vi "Redetection_Final EVT OUT.vi"(4 "Sweep # IN":i32, 5 "Detected event (1D)":cluster{dbl[][]}[](array[cluster]), 6 "EVT # (redetected)":i32, 7 "Number of event IN":i32[][](array[numeric])) -> (1 "Final EVT OUT":dbl[][](array[numeric]), 3 "Distribution (output)":T1)   [LabVIEW 2017]
uses:
  <vilib>/Analysis/NI_AALPro.lvlib
  <vilib>/Analysis/NI_AALBase.lvlib
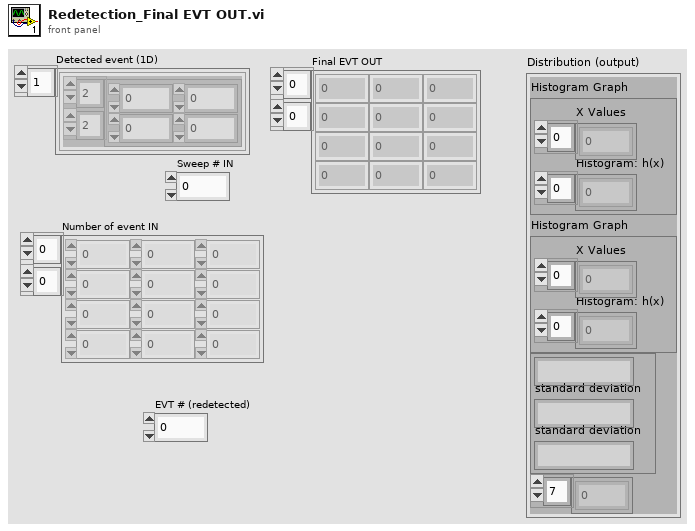
[diagram p1: front panel]
types:
  T1 = cluster{"Histogram Graph":cluster{"X Values":dbl[], "Histogram: h(x)":i32[]}, "Histogram Graph":cluster{"X Values":dbl[], "Histogram: h(x)":i32[]}, cluster{string, "standard deviation":string, "standard deviation":string}, i32[]}
  T2 = cluster{string, "standard deviation":string, "standard deviation":string}
  T3 = cluster{"X Values":dbl[], "Histogram: h(x)":i32[]}
  T4 = cluster{"Histogram Graph":cluster{"X Values":dbl[], "Histogram: h(x)":i32[]}, "Histogram Graph":cluster{"X Values":dbl[], "Histogram: h(x)":i32[]}, cluster{string, "standard deviation":string, "standard deviation":string}, "Number of event IN":i32[]}
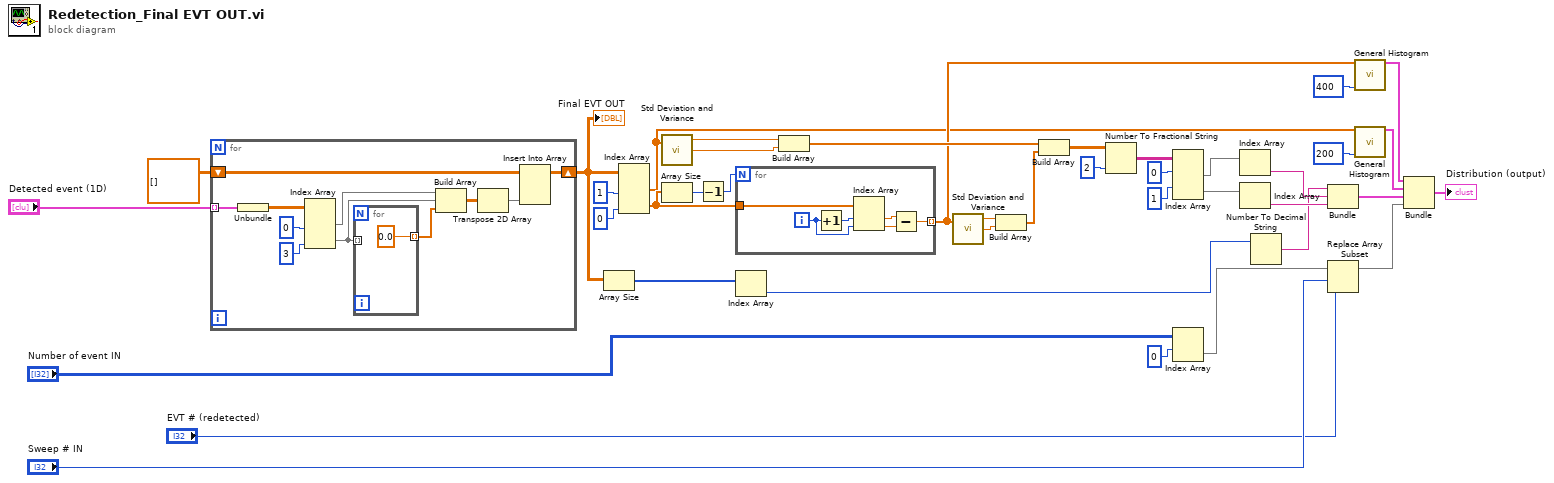
[diagram p0: block diagram]
diagram:
  n1 = for {
    tunnel: "Detected event (1D)" -> [w51] mode=indexing
    shift-right: [w46] -> w10
    shift-left: dbl[][] [] -> [w45]
    n2 = Unbundle(w51) -> (w50:dbl[][])
    n3 = Index Array(array=w50, index (col) #1=0 ("비활성화된 인덱스 (열)"), index (col) #2=3 ("인덱스 (열)")) -> (element #1=w47:dbl[], element #2=w44:dbl[])  [unwired: 2 in]
    n4 = for {
      tunnel: w44 -> [_] mode=indexing
      tunnel: [0.0] -> w43 mode=indexing
    }
    n5 = Build Array(w47, w44, w43) -> (w42:dbl[][])
    n6 = Transpose 2D Array(2D array=w42) -> (transposed array=w41:dbl[][])
    n7 = Insert Into Array(array=w45, new element=w41) -> (w46:dbl[][])  [unwired: 2 in]
  }
  "Final EVT OUT" <- w10
  n8 = Array Size(array=w10) -> (size(s)=w38:i32[])
  n9 = Index Array(array=w10, index (col) #1=1 ("비활성화된 인덱스 (열)"), index (col) #2=0 ("인덱스 (열)")) -> (element #1=w15:dbl[], element #2=w23:dbl[])  [unwired: 2 in]
  n10 = call <vilib>:"Std Deviation and Variance.vi"("X"=w15) -> ("mean"=w17:dbl, "standard deviation"=w18:dbl)  [unwired: 1 in, 1 out]
  n11 = Array Size(array=w23) -> (size(s)=w11:i32)
  n12 = Decrement(x=w11) -> (x-1=w12:i32)
  n13 = for {
    N: w12 -> [_]
    tunnel: w23 -> [w58]
    tunnel: [w53] -> w16 mode=indexing
    i -> [w56]
    n14 = Increment(x=w56) -> (x+1=w57:i32)
    n15 = Index Array(array=w58, index #1=w57, index #2=w56) -> (element #1=w55:dbl, element #2=w54:dbl)
    n16 = Subtract(x=w55, y=w54) -> (x-y=w53:dbl)
  }
  n17 = Index Array(array=w38) -> (element=w7:i32)  [unwired: 1 in]
  n18 = Build Array(w17, w18) -> (w22:dbl[])
  n19 = call <vilib>:"Std Deviation and Variance.vi"("X"=w16) -> ("mean"=w20:dbl, "standard deviation"=w19:dbl)  [unwired: 1 in, 1 out]
  n20 = Build Array(w20, w19) -> (w21:dbl[])
  n21 = Build Array(w22, w21) -> (w24:dbl[][])
  n22 = Number To Fractional String(number=w24, precision (6)=i16 2 ("폭(-)")) -> (F-format string=w26:string[][])  [unwired: 2 in]
  n23 = Index Array(array=w26, index (row) #1=0 ("인덱스 (행)"), index (row) #2=1 ("인덱스 (행)")) -> (element #1=w29:string[], element #2=w30:string[])  [unwired: 2 in]
  n24 = Index Array(array="Number of event IN", index (row)=0 ("비활성화된 인덱스 (열)")) -> (element=w4:i32[])  [unwired: 1 in]
  n25 = Index Array(array=w29) -> (element=w32:string)  [unwired: 1 in]
  n26 = Index Array(array=w30) -> (element=w33:string)  [unwired: 1 in]
  n27 = Number To Decimal String(number=w7) -> (decimal integer string=w31:string)  [unwired: 1 in]
  n28 = Bundle(w31, "standard deviation"=w32, "standard deviation"=w33) -> (w36:T2)  [unwired: 1 in]
  n29 = Replace Array Subset(array=w4, new element="EVT # (redetected)", index="Sweep # IN") -> (w3:i32[])
  n30 = call <vilib>:"General Histogram.vi"("X"=w16, "# bins"=400) -> ("Histogram Graph"=w34:T3)  [unwired: 9 in, 4 out]
  n31 = call <vilib>:"General Histogram.vi"("X"=w15, "# bins"=200) -> ("Histogram Graph"=w35:T3)  [unwired: 9 in, 4 out]
  n32 = Bundle("Histogram Graph"=w34, "Histogram Graph"=w35, w36, "Number of event IN"=w3) -> (→"Distribution (output)":T4)  [unwired: 1 in]
